vi "LogDBCreateRef.vi"(8 "error in (no error)":errorcluster, 9 "db":bool, 10 "Pfad in":path=path "C:/Git/B2G/B2G_db_rz.dsn", 11 "Refnum in":T1) -> (0 "error out":errorcluster, 3 "Refnum out":T1)   [LabVIEW 2011]
uses:
  <vilib>/addons/database/Connection.llb/Conn ObjectReference.ctl
  <vilib>/addons/database/Connection.llb/DB Tools Open Connec (Path).vi
  <vilib>/addons/database/NI_Database_API.lvlib
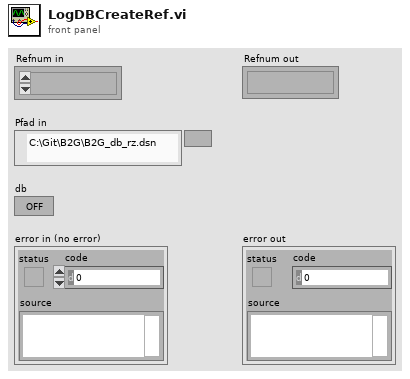
[diagram p1: front panel]
types:
  T1 = typedef "NI_Database_API.lvlib/Conn ObjectReference.ctl" = refnum<k1>
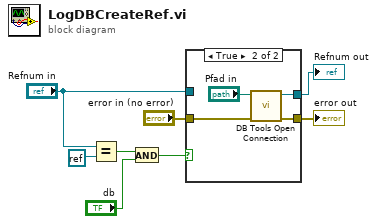
[diagram p0: block diagram]
diagram:
  n1 = Equal?(x="Refnum in", y=refnum<k0> refnum) -> (x = y?=w1:bool)
  n2 = And(x=w1, y="db") -> (x .and. y?=w2:bool)
  n3 = case shown="True" w2 {
    tunnel: [w9 w12] -> w7
    tunnel: [w10 w14] -> w6
    tunnel: "error in (no error)" -> [w10 w13]
    tunnel: "Refnum in" -> [w9 _]
    frame False {
    }
    frame True {
      n4 = call-poly <vilib>:"DB Tools Open Connection.vi"("error in (no error)"=w13, "connection information"="Pfad in") -> ("error out"=w14:errorcluster, "connection reference"=w12:T1)  [unwired: 6 in]
    }
  }
  "Refnum out" <- w7
  "error out" <- w6
